vi "H5Oget_info_by_name.vi"(6 "error in (no error)":errorcluster, 7 "lapl_id":T1, 8 "Name":string, 9 "HDF5 Ref":T1) -> (0 "error out":errorcluster, 2 "Object Info":T2 {"H5O_hdr_info_t"."mesg"."shared" format="%.0x"; "H5O_hdr_info_t"."mesg"."present" format="%.0x"; "H5O_hdr_info_t"."flags" format="%.0x"; "type" items=["H5O_TYPE_UNKNOWN"=-1, "H5O_TYPE_GROUP"=0, "H5O_TYPE_DATASET"=1, "H5O_TYPE_NAMED_DATATYPE"=2]}, 3 "HDF5 Ref out":T1)   [LabVIEW 2017]
doc: "Retrieves the metadata for an object, identifying the object by \n location and relative name."
uses:
  <vilib>/UPVI/lvhdf5/library.llb/HDF5 Ref.ctl
  <vilib>/UPVI/lvhdf5/object.llb/LVH5O_info_t.ctl
  <vilib>/UPVI/lvhdf5/object.llb/H5O_type_t.ctl
  <vilib>/UPVI/lvhdf5/object.llb/H5O_hdr_info_t.ctl
  <vilib>/UPVI/lvhdf5/library.llb/H5_ih_info_t.ctl
  <vilib>/UPVI/lvhdf5/object.llb/H5O_info_t.ctl
  <vilib>/UPVI/lvhdf5/hdf5.dll
panel:
  # "LVHDF5 Toolkit\nCopyright (c) 2005-2013 by Jason D. Sommerville\nCopyright (c) 2014 by UPVI, LLC.\n\nThis use and distribution of this file is governed by the terms found in \nLICENSE.txt distributed with this toolkit and installed at\n <user.lib>\\_lvhdf5\\LICENSE.txt"
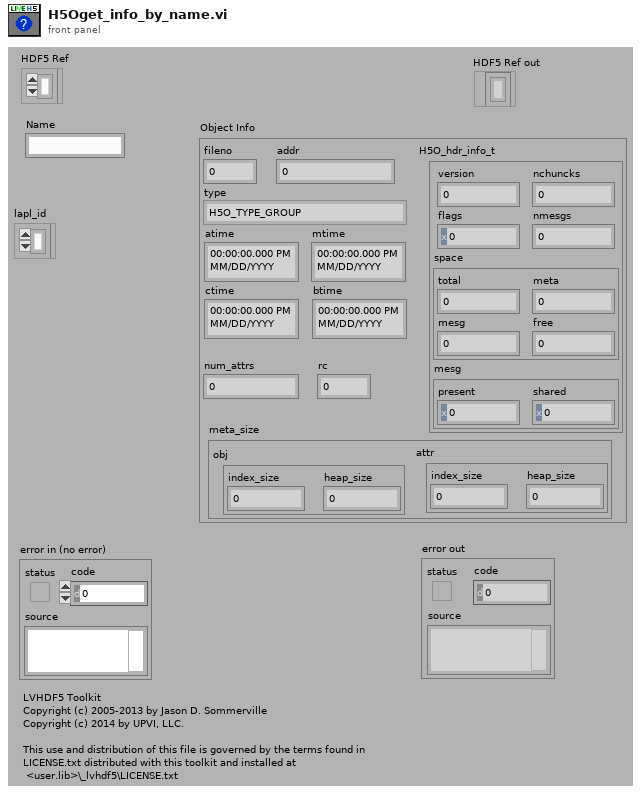
[diagram p1: front panel]
types:
  T1 = typedef "HDF5 Ref.ctl" = refnum<k1>
  T2 = typedef "LVH5O_info_t.ctl" = cluster{"fileno":u32, "addr":u64, "type":T3, "rc":u32, "atime":timestamp, "mtime":timestamp, "ctime":timestamp, "btime":timestamp, "num_attrs":i64, "H5O_hdr_info_t":T4, "meta_size":cluster{"obj":T5, "attr":T5}}
  T3 = typedef "H5O_type_t.ctl" = i32
  T4 = typedef "H5O_hdr_info_t.ctl" = cluster{"version":u32, "nmesgs":u32, "nchuncks":u32, "flags":u32, "space":cluster{"total":u64, "meta":u64, "mesg":u64, "free":u64}, "mesg":cluster{"present":u64, "shared":u64}}
  T5 = typedef "H5_ih_info_t.ctl" = cluster{"index_size":u64, "heap_size":u64}
  T6 = typedef "H5O_info_t.ctl" = cluster{"fileno":u32, "unused":u32, "addr":u64, "type":T3, "rc":u32, "atime":i64, "mtime":i64, "ctime":i64, "btime":i64, "num_attrs":i64, "H5O_hdr_info_t":T4, "meta_size":cluster{"obj":T5, "attr":T5}}
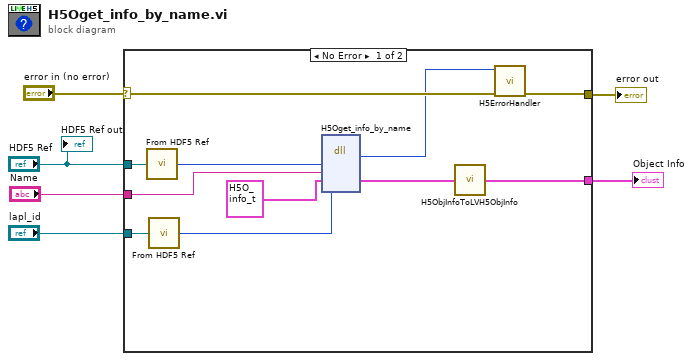
[diagram p0: block diagram]
diagram:
  n1 = case shown="No Error" "error in (no error)" {
    selector: "error in (no error)" -> [w17 w18]
    tunnel: [w16 w18] -> w5
    tunnel: "HDF5 Ref" -> [w15 _]
    tunnel: "Name" -> [w12 _]
    tunnel: [w8 _] -> w1
    tunnel: "lapl_id" -> [w11 _]
    frame No Error {
      n2 = call <vilib>:"From HDF5 Ref.vi"("HDF5 Ref"=w15) -> ("I32"=w14:i32)
      n3 = call <vilib>:"From HDF5 Ref.vi"("HDF5 Ref"=w11) -> ("I32"=w10:i32)
      n4 = dll-call lib="C:/Program Files/National Instruments/LabVIEW 2017/vi.lib/UPVI/lvhdf5/hdf5.dll" fn="H5Oget_info_by_name"("loc_id"=w14, "object_name"=w12, "info"=T6 {"fileno"=0, "unused"=0, "addr"=0, "type"=0, "rc"=0, "atime"=0, "mtime"=0, "ctime"=0, "btime"=0, "num_attrs"=0, "H5O_hdr_info_t"={"version"=0, "nmesgs"=0, "nchuncks"=0, "flags"=0, "space"={"total"=0, "meta"=0, "mesg"=0, "free"=0}, "mesg"={"present"=0, "shared"=0}}, "meta_size"={"obj"={"index_size"=0, "heap_size"=0}, "attr"={"index_size"=0, "heap_size"=0}}} ("H5O_info_t"), "lapl_id"=w10) -> ("return type"=w13:i32, "info"=w9:T6)  [unwired: 6 in, 2 out]
      n5 = call <vilib>:"H5ObjInfoToLVH5ObjInfo.vi"("H5O_info_t"=w9) -> ("LVH5O_info_t"=w8:T2)
      n6 = call <vilib>:"H5ErrorHandler.vi"("error in (no error)"=w17, "herr_t"=w13) -> ("error out"=w16:errorcluster)  [unwired: 3 in, 4 out]
    }
    frame Error {
    }
  }
  "error out" <- w5
  "Object Info" <- w1
  "HDF5 Ref out" <- "HDF5 Ref"
